vi "WPI_SwitchClose.vi"(8 "error in (no error)":errorcluster, 11 "SwitchDevRef":T1={"DevStatus"={"status"=FALSE, "code"=0, "source"=""}, "DIO Channel"=enum."Invalid", "CntIndex"=enum."Invalid", "Normally Closed"=FALSE}) -> (0 "error out":errorcluster)   [LabVIEW 2017]
doc: "Returns the value of the digital input that you specify.\n\nThis software is licensed. Open the labview\\readme\\WPI Robotics Library Open Source License.txt file for more information."
uses:
  <vilib>/Rock Robotics/WPI/Switch/WPI_SwitchDevRef.ctl
  <vilib>/Rock Robotics/SystemInterfaces/DIO/FPGA_DIOChannel.ctl
  <vilib>/Rock Robotics/SystemInterfaces/Counter/FPGA_CounterCtrSystemIndex.ctl
  <vilib>/Rock Robotics/WPI/DigitalInput/WPI_DigitalInputDevRef.ctl
  <vilib>/Rock Robotics/WPI/Counter/WPI_CounterDevRef.ctl
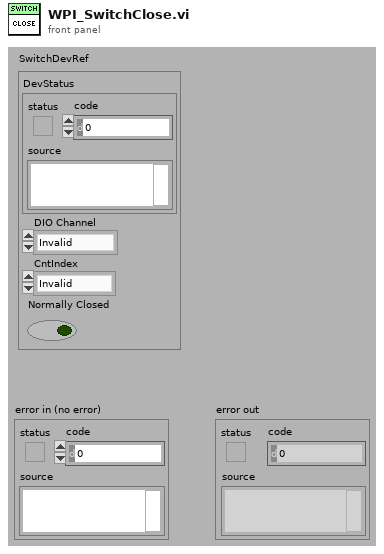
[diagram p1: front panel]
types:
  T1 = typedef "WPI_SwitchDevRef.ctl" = cluster{"DevStatus":errorcluster, "DIO Channel":T2, "CntIndex":T3, "Normally Closed":bool}
  T2 = typedef "FPGA_DIOChannel.ctl" = enum8{"DIO 0", "DIO 1", "DIO 2", "DIO 3", "DIO 4", "DIO 5", "DIO 6", "DIO 7", "DIO 8", "DIO 9", "DIO MXP 0", "DIO MXP 1", "DIO MXP 2", "DIO MXP 3", "DIO MXP 4", "DIO MXP 5", "DIO MXP 6", "DIO MXP 7", "DIO MXP 8", "DIO MXP 9", "DIO MXP 10", "DIO MXP 11", "DIO MXP 12", "DIO MXP 13", "DIO MXP 14", "DIO MXP 15", "SPI Port CS1", "SPI Port CS2", "SPI Port CS3", "SPI Port MISO", "SPI Port MOSI", "Invalid"}
  T3 = typedef "FPGA_CounterCtrSystemIndex.ctl" = enum8{"Ctr 0", "Ctr 1", "Ctr 2", "Ctr 3", "Ctr 4", "Ctr 5", "Ctr 6", "Ctr 7", "Invalid"}
  T4 = typedef "WPI_DigitalInputDevRef.ctl" = cluster{"DevStatus":errorcluster, "DIO Channel":T2}
  T5 = typedef "WPI_CounterDevRef.ctl" = cluster{"DevStatus":errorcluster, "CntIndex":T3}
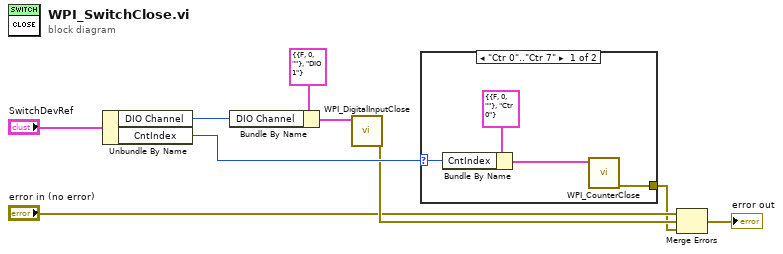
[diagram p0: block diagram]
diagram:
  n1 = Unbundle By Name("SwitchDevRef") -> ("DIO Channel"=w8:T2, "CntIndex"=w5:T3)
  n2 = Bundle By Name(cluster=T4 {"DevStatus"={"status"=FALSE, "code"=0, "source"=""}, "DIO Channel"=enum."DIO 1"} ("DigitalInputDevRef"), "DIO Channel"=w8) -> (w6:T4)
  n3 = call <vilib>:"WPI_DigitalInputClose.vi"("DigitalInputDevRef"=w6) -> ("error out"=w4:errorcluster)  [unwired: 10 in]
  n4 = case shown="\"Ctr 0\"..\"Ctr 7\"" w5 {
    selector: w5 -> [w12 _]
    tunnel: [w11 _] -> w2
    frame "Ctr 0".."Ctr 7" {
      n5 = Bundle By Name(cluster=T5 {"DevStatus"={"status"=FALSE, "code"=0, "source"=""}, "CntIndex"=enum."Ctr 0"} ("CounterDevRef in"), "CntIndex"=w12) -> (w10:T5)
      n6 = call <vilib>:"WPI_CounterClose.vi"("CounterDevRef"=w10) -> ("error out"=w11:errorcluster)  [unwired: 10 in]
    }
    frame "Invalid" {
      # "If switch was used for Limit, there will be no counter used."
    }
  }
  n7 = Merge Errors("error in (no error)", w4, w2) -> (→"error out":errorcluster)
